vi "Untitled 3.vi"() -> ()   [LabVIEW 2012]
uses:
  <vilib>/DAQmx/write.llb/DAQmx Write (Digital U8 1Chan 1Samp).vi
  <vilib>/DAQmx/create/channels.llb/DAQmx Create Channel (DO-Digital Output).vi
  <vilib>/DAQmx/miscellaneous.llb/DAQmx Fill In Error Info.vi
  <resource>/objmgr/daqmx.rc
panel:
  out "number of samples written per channel":u32
  in  "data 2":u8
  in  "data":bool
  in  "Array":bool[](array[boolean])
  in  "DO.OutputDriveType":i32(ring)=12573 items=["Active Drive"=12573, "Open Collector"=12574]
  in  "Stop Button":bool
  out "error out":errorcluster
  in  "lines":tag
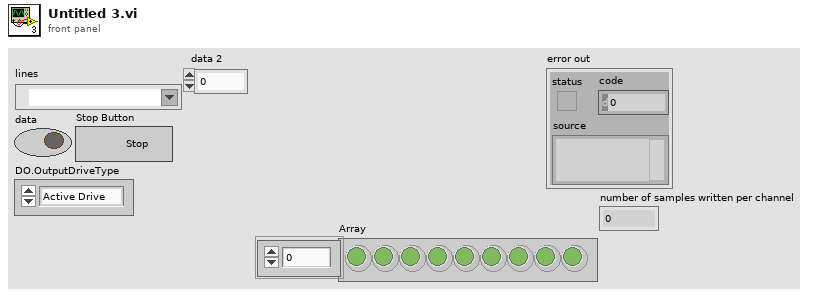
[diagram p1: front panel]
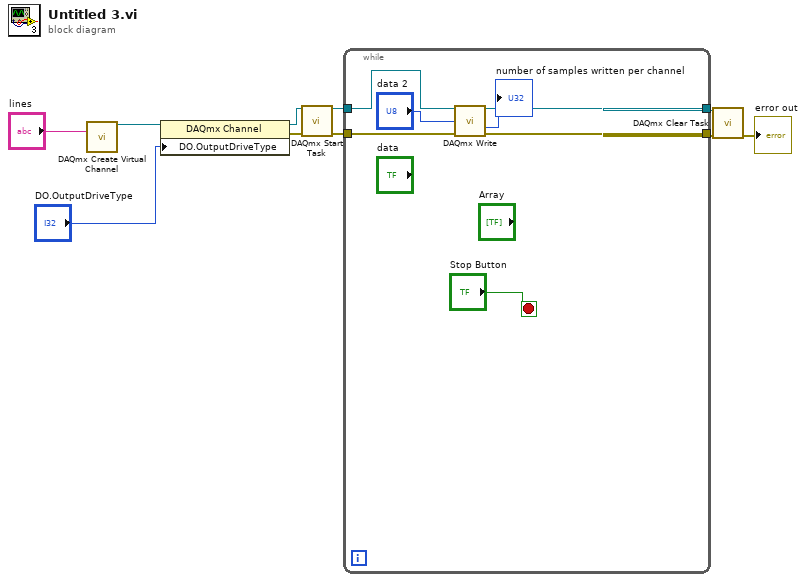
[diagram p0: block diagram]
diagram:
  n1 = call-poly <vilib>:"DAQmx Create Virtual Channel.vi"("lines"="lines") -> ("task out"=w8:refnum<k21>)  [unwired: 13 in, 1 out]
  n2 = property class="DAQmx Channel"(reference=w8, "DO.OutputDriveType"="DO.OutputDriveType") -> (reference out=w6:refnum<k21>, error out=w5:errorcluster)  [unwired: 1 in]
  n3 = call <vilib>:"DAQmx Start Task.vi"("task/channels in"=w6, "error in"=w5) -> ("task out"=w4:refnum<k21>, "error out"=w3:errorcluster)  [unwired: 12 in]
  n4 = while {
    tunnel: w4 -> [w14]
    tunnel: w3 -> [w16]
    tunnel: [w15] -> w2
    tunnel: [w13] -> w1
    stop <- "Stop Button" stop-if-true
    n5 = call-poly <vilib>:"DAQmx Write.vi"("task/channels in"=w14, "data"="data 2", "error in"=w16) -> ("task out"=w13:refnum<k21>, "number of samples written per channel"=→"number of samples written per channel":u32, "error out"=w15:errorcluster)  [unwired: 10 in]
  }
  n6 = call <vilib>:"DAQmx Clear Task.vi"("task in"=w1, "error in"=w2) -> ("error out"=→"error out":errorcluster)  [unwired: 13 in]
